vi "SMU current sweep one measurement (SubVI).vi"(5 "Timeout (Sec)":dbl, 6 "Channel Name":string, 7 "Current Level End":dbl, 8 "error in (no error)":errorcluster, 9 "Current Level Start":dbl, 10 "Points to average":i32, 11 "IVI Refnum in":refnum<k15>) -> (0 "error out":errorcluster, 1 "Average voltage":dbl, 3 "IVI Refnum out":refnum<k15>, 4 "Average current":dbl)   [LabVIEW 2017]
uses:
  <instrlib>/niDCPower/nidcpower.llb/niDCPower Wait For Event - Event.ctl
panel:
  out "average resistance":dbl
  out "output cluster":T1
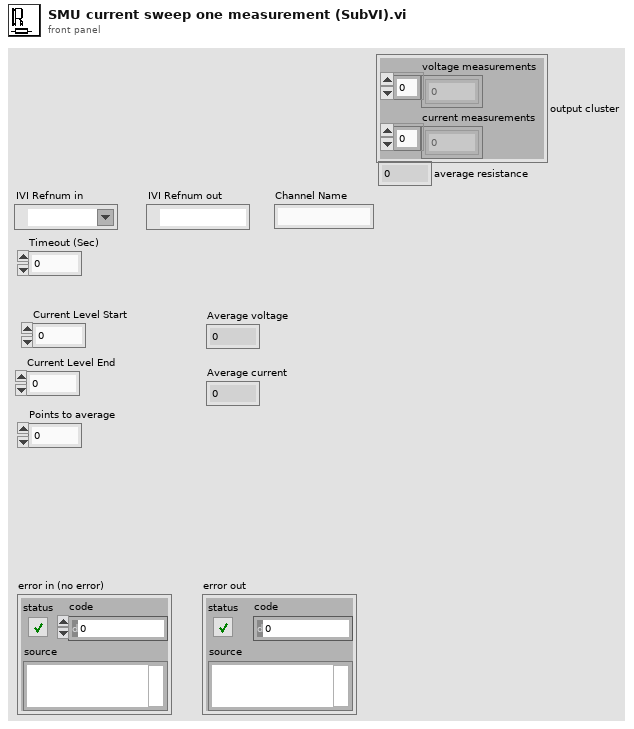
[diagram p1: front panel]
types:
  T1 = cluster{"voltage measurements":dbl[], "current measurements":dbl[]}
  T2 = typedef "niDCPower Wait For Event - Event.ctl" = i32
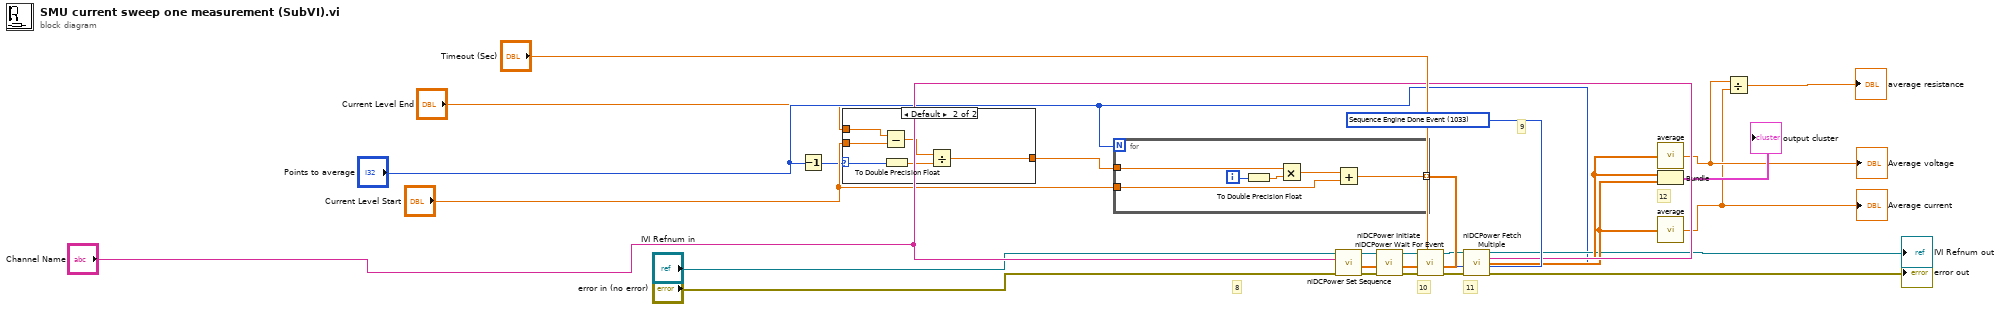
[diagram p0: block diagram]
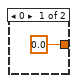
[diagram p2: hidden frame]
diagram:
  w22 = T2 1033 items=["Source Complete Event"=1030, "Measure Complete Event"=1031, "Sequence Iteration Complete Event"=1032, "Sequence Engine Done Event"=1033, "Pulse Complete Event"=1051, "Ready For Pulse Trigger Event"=1052] ("event")
  # "10"
  # "8"
  # "9"
  # "12"
  # "11"
  n1 = Decrement(x="Points to average") -> (x-1=w5:i32)
  n2 = case shown="Default" w5 {
    selector: w5 -> [_ w27]
    tunnel: "Current Level End" -> [_ w32]
    tunnel: [0.0 w30] -> w6
    tunnel: "Current Level Start" -> [_ w28]
    frame 0 {
    }
    frame Default {
      n3 = Subtract(x=w32, y=w28) -> (x-y=w31:dbl)
      n4 = To Double Precision Float(number=w27) -> (double precision float=w29:dbl)
      n5 = Divide(x=w31, y=w29) -> (x/y=w30:dbl)
    }
  }
  n6 = for {
    N: "Points to average" -> [_]
    tunnel: w6 -> [w38]
    tunnel: "Current Level Start" -> [w35]
    tunnel: [w33] -> w25 mode=indexing
    i -> [w37]
    n7 = To Double Precision Float(number=w37) -> (double precision float=w34:dbl)
    n8 = Multiply(x=w38, y=w34) -> (x*y=w36:dbl)
    n9 = Add(x=w36, y=w35) -> (x+y=w33:dbl)
  }
  n10 = call <instrlib>:"niDCPower Set Sequence.vi"("error in (no error)"="error in (no error)", "values"=w25, "channel name"="Channel Name", "instrument handle"="IVI Refnum in") -> ("error out"=w17:errorcluster, "instrument handle out"=w16:refnum<k15>)  [unwired: 1 in, 5 out]
  n11 = call <instrlib>:"niDCPower Initiate.vi"("error in (no error)"=w17, "instrument handle"=w16) -> ("error out"=w19:errorcluster, "instrument handle out"=w18:refnum<k15>)  [unwired: 8 out]
  n12 = call <instrlib>:"niDCPower Wait For Event.vi"("timeout (sec)"="Timeout (Sec)", "error in (no error)"=w19, "event"=w22, "instrument handle"=w18) -> ("error out"=w23:errorcluster, "instrument handle out"=w24:refnum<k15>)  [unwired: 6 out]
  n13 = call <instrlib>:"niDCPower Fetch Multiple.vi"("instrument handle"=w24, "channel name"="Channel Name", "count (1)"="Points to average", "error in (no error)"=w23) -> ("instrument handle out"=→"IVI Refnum out":refnum<k15>, "voltage measurements"=w13:dbl[], "current measurements"=w12:dbl[], "error out"=→"error out":errorcluster)  [unwired: 1 in, 7 out]
  n14 = call "average.vi"("Array"=w13) -> ("Average"=w3:dbl)
  "Average voltage" <- w3
  n15 = Bundle("voltage measurements"=w13, "current measurements"=w12) -> (→"output cluster":T1)  [unwired: 1 out]
  n16 = call "average.vi"("Array"=w12) -> ("Average"=w2:dbl)
  "Average current" <- w2
  n17 = Divide(x=w3, y=w2) -> (x/y=→"average resistance":dbl)
